vi "Pipelined Burst FFT Core FXP.vi"(9 "xn_im":fxp<+,16,1>, 10 "xn_re":fxp<+,16,1>, 11 "FFT State Info In":T2) -> (0 "Output Valid":bool, 2 "FFT Output":T1, 4 "xk_index":fxp<+,9,9>, 6 "edone":bool)   [LabVIEW 2011]
uses:
  <vilib>/rvi/IPIntegrationNode/IPINode_Utilities/niFpgaIPINodeSimCore.vi
  <vilib>/rvi/FXPMathLib/basic elements/FxpDiscreteDelay/XNode/nifxpmath_DiscreteDelay.xnode
  <vilib>/rvi/XilinxIP/XIPIN_XNode/niFpgaXIPIN.xnode
  <userlib>/FPGA Library/Code Development/Signal Processing/FFT Block/FFT/FFT Process/Fast Fourier Transform/FastFourierTransform_F1A05D14459132E02A085DB04D52F246.dll
  <vilib>/rvi/IPIntegrationNode/IPINode_Xnode/niFpgaIPINode.xnode
panel:
  out "xk_re":fxp<+,32,32>
  out "xk_im":fxp<+,32,32>
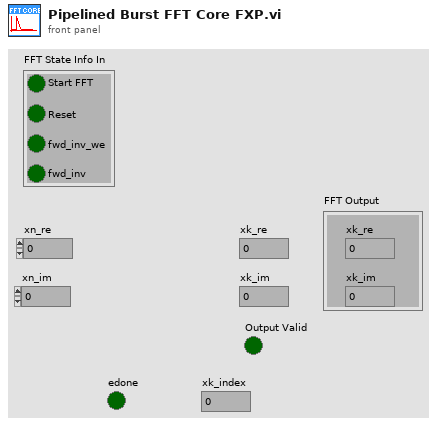
[diagram p1: front panel]
types:
  T1 = cluster{"xk_im":fxp<+,32,32>, "xk_re":fxp<+,32,32>}
  T2 = cluster{"Reset":bool, "Start FFT":bool, "fwd_inv_we":bool, "fwd_inv":bool}
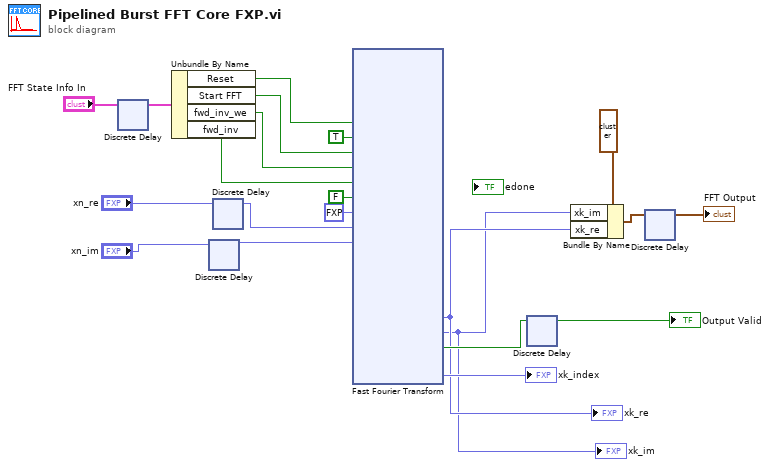
[diagram p0: block diagram]
diagram:
  n1 = xnode "Discrete Delay"("D"="FFT State Info In") -> ("Q"=w16:T2)
  n2 = Unbundle By Name(w16) -> ("Reset"=w13:bool, "Start FFT"=w11:bool, "fwd_inv_we"=w10:bool, "fwd_inv"=w9:bool)
  n3 = xnode "Discrete Delay"("D"="xn_im") -> ("Q"=w7:fxp<+,16,1>)
  n4 = xnode "Discrete Delay"("D"="xn_re") -> ("Q"=w8:fxp<+,16,1>)
  n5 = xnode ("Fast Fourier Transform")("sclr"=w13, "ce"=TRUE, "start"=w11, "fwd_inv_we"=w10, "fwd_inv"=w9, "scale_sch_we"=FALSE, "scale_sch"=fxp<+,10,10> 0.0, "xn_re"=w8, "xn_im"=w7) -> ("xk_re"=w2:fxp<+/-,16,1>, "xk_im"=w1:fxp<+/-,16,1>, "dv"=w6:bool, "xk_index"=→"xk_index":fxp<+,10,10>)  [unwired: 5 out]
  "xk_im" <- w1
  "xk_re" <- w2
  n6 = xnode "Discrete Delay"("D"=w6) -> ("Q"=→"Output Valid":bool)
  n7 = Bundle By Name(cluster=T1 {"xk_im"=0.0, "xk_re"=0.0} ("FFT Output"), "xk_im"=w1, "xk_re"=w2) -> (w17:T1)
  n8 = xnode "Discrete Delay"("D"=w17) -> ("Q"=→"FFT Output":T1)
